vi "Multistage Decimation Filter Design.vi"() -> ()   [LabVIEW 2023]
doc: "Demonstrates how to use the DFD NStage MRate Filter Design VI to design a decimation filter with a large factor and use the DFD Plot NStage MRate Freq Response VI to analyze the decimation filter.\n\nComplete the following steps to use this VI.\n1) Run the VI.\n2) Observe the Magnitude Responses graph.\n3) Examine the controls to learn how to set the specifications."
uses:
  <vilib>/addons/Digital Filter Design/_Objects.llb/DFD Multirate Filter Specification (Design).ctl
  <vilib>/addons/Digital Filter Design/_Objects.llb/DFD Filter Ripple Specification (Design).ctl
  <vilib>/addons/Digital Filter Design/_Objects.llb/DFD Multirate Filtering Mode.ctl
  <vilib>/addons/Digital Filter Design/NI_DigFilterLicensed.lvlib
panel:
  out "Error Message":string
  in  "Factor":i32=50
  in  "Manual Factorization":i32[](array[numeric])=[10, 5]
  in  "Input Sampling Frequency [Hz]":dbl=100000.0
  out "Magnitude Responses":cluster{"f0":dbl, "df":dbl, "values":dbl[]}[](graph)
  in  "Ripple Specifications":T1={"passband"=0.01, "stopband"=0.001, "dB/linear? (T: dB)"=FALSE}
  in  "Frequency Specifications [Hz]":T2={"fpass"=100.0, "fstop"=800.0}
  # "Select Help>>Show Context Help and move the cursor over the VI icon for more information."
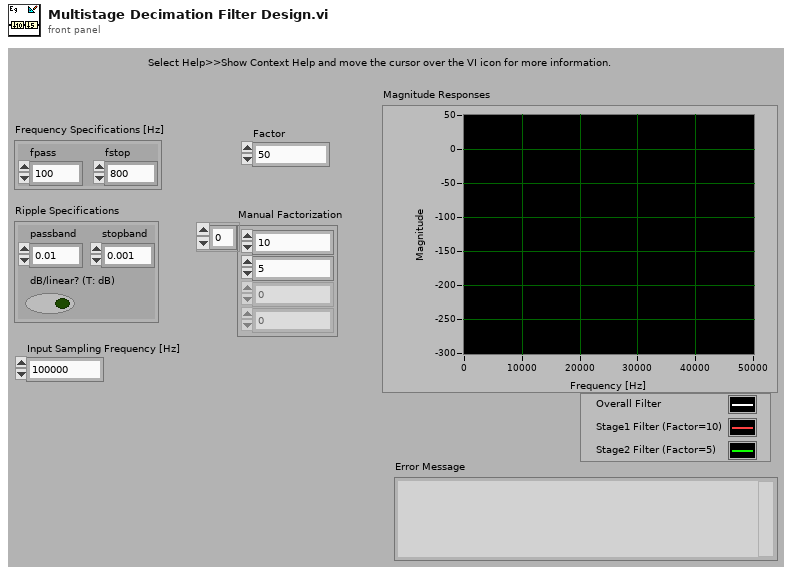
[diagram p1: front panel]
types:
  T1 = typedef "NI_DigFilterLicensed.lvlib/DFD Filter Ripple Specification (Design).ctl" = cluster{"passband":dbl, "stopband":dbl, "dB/linear? (T: dB)":bool}
  T2 = typedef "NI_DigFilterLicensed.lvlib/DFD Multirate Filter Specification (Design).ctl" = cluster{"fpass":dbl, "fstop":dbl}
  T3 = typedef "NI_DigFilterLicensed.lvlib/DFD Multirate Filtering Mode.ctl" = u16
  T4 = typedef "NI_DigFilterLicensed.lvlib/DFD Multirate Filter Obj.ctl" = cluster{"mMRate_Structure":enum16{"CIC", "FIR", "IIR", "Lattice"}, "mMRate_Mode":T5, "mMRate_Factor":i32, "mMRate_FIRParams":cluster{"mMRate_FIR_H":dbl[], "mMRate_FIR_IsNyquist?":bool, "mMRate_FIR_IsSymmetric?":bool}, "mMRate_CICParams":cluster{"mMRate_CIC_#Stage":i32, "mMRate_CIC_Lag":i32, "mMRate_CIC_Type":enum16{"Lowpass", "Highpass"}}, "mMRate_Order":i32, "mMRate_Version":string, "mMRate_Comments":string, "mMRate_RationalFactor":cluster{"mMRate_L":i32, "mMRate_M":i32}, "mMRate_Fs":dbl, "mMRate_Quantized?":bool, "mMRate_QFilterGain":dbl, "mMRate_CoefWl":i16, "mMRate_Scaling":cluster{"mMRate_ScaleByPowerOf2?":bool, "mMRate_ScaleType":T6}, "mMRate_InputWl":i16, "mMRate_OutputWl":i16, "mMRate_OutputMode":T7, "mMRate_MultMode":T8, "mMRate_BitPruning":bool, "mMRate_GainWl":i16, "mMRate_OutputFwl":i16, "mMRate_SumIwl":i16, "mMRate_InputIwl ":i16, "mMRate_SumWl":i16, "mMRate_CoefIwl":i16}
  T5 = typedef "NI_DigFilterLicensed.lvlib/DFD Multirate Mode.ctl" = i16
  T6 = typedef "NI_DigFilterLicensed.lvlib/DFD Coef Norm Type.ctl" = enum16{"No Norm", "Time Domain 1-Norm", "Time Domain 2-Norm", "Time Domain Inf-Norm"}
  T7 = typedef "NI_DigFilterLicensed.lvlib/DFD Round-off Mode.ctl" = enum16{"Nearest", "Truncation"}
  T8 = typedef "NI_DigFilterLicensed.lvlib/DFD FXP MRate Multiply Mode.ctl" = enum16{"Truncated", "Full"}
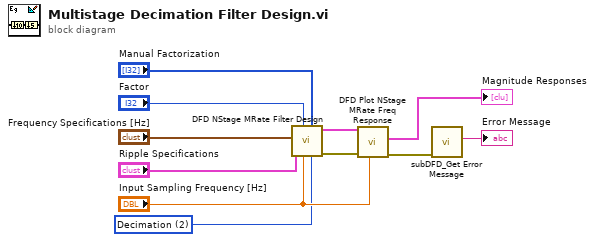
[diagram p0: block diagram]
diagram:
  w3 = T3 2 items=["No Rate Change", "Interpolation", "Decimation"] ("Filtering Mode")
  n1 = call <vilib>:"DFD NStage MRate Filter Design.vi"("filtering mode"=w3, "manual factorization"="Manual Factorization", "fs in [Hz]"="Input Sampling Frequency [Hz]", "factor"="Factor", "ripple specs"="Ripple Specifications", "freq specs [Hz]"="Frequency Specifications [Hz]") -> ("error out"=w5:errorcluster, "multirate filters out"=w9:T4[])  [unwired: 2 in, 2 out]
  n2 = call <vilib>:"DFD Plot NStage MRate Freq Response.vi"("fs in [Hz]"="Input Sampling Frequency [Hz]", "error in (no error)"=w5, "multirate filters in"=w9) -> ("error out"=w1:errorcluster, "magnitude responses"=→"Magnitude Responses":cluster{"f0":dbl, "df":dbl, "values":dbl[]}[])  [unwired: 4 in, 3 out]
  n3 = call <vilib>:"subDFD_Get Error Message.vi"("error in (no error)"=w1) -> ("Error Message"=→"Error Message":string)  [unwired: 10 out]
